vi "Auto 7.vi"(8 "Error In":errorcluster) -> (0 "Error Out":errorcluster)   [LabVIEW 2014]
uses:
  <vilib>/Rock Robotics/WPI/Solenoid/WPI_SolenoidValue.ctl
  <vilib>/Rock Robotics/WPI/Solenoid/WPI_SolenoidSetEnum.vi
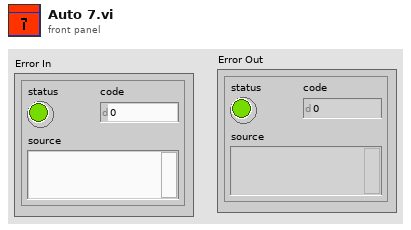
[diagram p1: front panel]
types:
  T1 = typedef "WPI_SolenoidValue.ctl" = enum16{"Off", "On", "Forward", "Reverse"}
  T2 = typedef "WPI_SolenoidDevRef.ctl" = cluster{"DevStatus":errorcluster, "Pneumatics Control Module":u8, "Forward Solenoid Channel":T3, "Reverse Solenoid Channel":T3}
  T3 = typedef "WPI_SolenoidChannel.ctl" = enum8{"Solenoid 0", "Solenoid 1", "Solenoid 2", "Solenoid 3", "Solenoid 4", "Solenoid 5", "Solenoid 6", "Solenoid 7", "Invalid"}
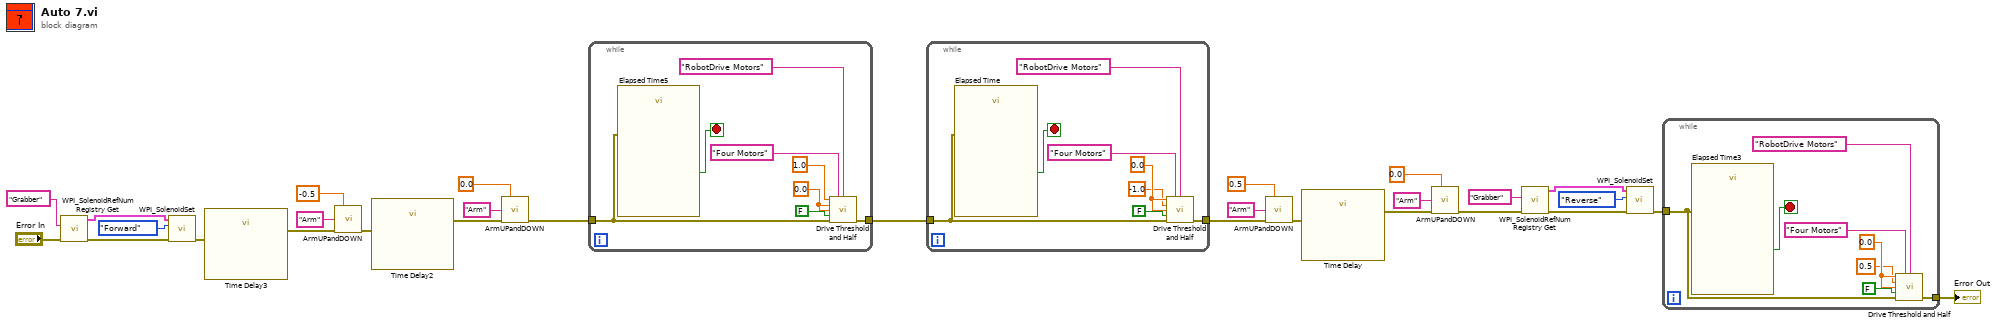
[diagram p0: block diagram]
diagram:
  n1 = call <vilib>:"WPI_SolenoidRefNum Registry Get.vi"("error in (no error)"="Error In", "refnum name"="Grabber") -> ("error out"=w16:errorcluster, "SolenoidDevRef"=w17:T2)  [unwired: 8 in]
  n2 = call-poly <vilib>:"WPI_SolenoidSet.vi"("error in (no error)"=w16, "Value"=WPI_SolenoidValue."Forward", "SolenoidDevRef"=w17) -> ("error out"=w5:errorcluster)  [unwired: 7 in, 1 out]
  n3 = call "Time Delay3"("error in (no error)"=w5) -> ("error out"=w4:errorcluster)  [unwired: 10 in]
  n4 = call "ArmUPandDOWN.vi"("Arm Value"=-0.5, "Arm"="Arm" ("refnum name"), "Error In"=w4) -> ("Error Out"=w27:errorcluster)  [unwired: 12 in]
  n5 = call "Time Delay2"("error in (no error)"=w27) -> ("error out"=w10:errorcluster)  [unwired: 10 in]
  n6 = call "ArmUPandDOWN.vi"("Arm Value"=0.0, "Arm"="Arm" ("refnum name"), "Error In"=w10) -> ("Error Out"=w3:errorcluster)  [unwired: 12 in]
  n7 = while {
    tunnel: w3 -> [w32]
    tunnel: [w34] -> w2
    stop <- w33 stop-if-true
    w30 = 0.0 ("X In")
    n8 = call "Elapsed Time5"("error in (no error)"=w32) -> ("Time has Elapsed"=w33:bool)  [unwired: 11 in, 7 out]
    n9 = call "Drive Threshold and Half.vi"("X In"=1.0 ("Arm Value"), "Drive refnum name"="Four Motors" ("refnum name"), "Send to DB Name"="RobotDrive Motors" ("Name"), "Y In"=w30, "R In"=w30, "Speed Toggle"=FALSE ("Grabber Open/Close"), "Error In"=w32) -> ("Error Out"=w34:errorcluster)  [unwired: 8 in]
  }
  n10 = while {
    tunnel: w2 -> [w38]
    tunnel: [w42] -> w1
    stop <- w39 stop-if-true
    w41 = 0.0 ("Arm Value")
    n11 = call "Elapsed Time"("error in (no error)"=w38) -> ("Time has Elapsed"=w39:bool)  [unwired: 11 in, 7 out]
    n12 = call "Drive Threshold and Half.vi"("X In"=w41, "Drive refnum name"="Four Motors" ("refnum name"), "Send to DB Name"="RobotDrive Motors" ("Name"), "Y In"=-1.0 ("X In"), "R In"=w41, "Speed Toggle"=FALSE ("Grabber Open/Close"), "Error In"=w38) -> ("Error Out"=w42:errorcluster)  [unwired: 8 in]
  }
  n13 = call "ArmUPandDOWN.vi"("Arm Value"=0.5, "Arm"="Arm" ("refnum name"), "Error In"=w1) -> ("Error Out"=w25:errorcluster)  [unwired: 12 in]
  n14 = call "Time Delay"("error in (no error)"=w25) -> ("error out"=w7:errorcluster)  [unwired: 10 in]
  n15 = call "ArmUPandDOWN.vi"("Arm Value"=0.0, "Arm"="Arm" ("refnum name"), "Error In"=w7) -> ("Error Out"=w6:errorcluster)  [unwired: 12 in]
  n16 = call <vilib>:"WPI_SolenoidRefNum Registry Get.vi"("error in (no error)"=w6, "refnum name"="Grabber") -> ("error out"=w21:errorcluster, "SolenoidDevRef"=w22:T2)  [unwired: 8 in]
  n17 = call-poly <vilib>:"WPI_SolenoidSet.vi"("error in (no error)"=w21, "Value"=WPI_SolenoidValue."Reverse", "SolenoidDevRef"=w22) -> ("error out"=w18:errorcluster)  [unwired: 7 in, 1 out]
  n18 = while {
    tunnel: w18 -> [w46]
    tunnel: [w50] -> w26
    stop <- w47 stop-if-true
    w49 = 0.0 ("Arm Value")
    n19 = call "Elapsed Time3"("error in (no error)"=w46) -> ("Time has Elapsed"=w47:bool)  [unwired: 11 in, 7 out]
    n20 = call "Drive Threshold and Half.vi"("X In"=w49, "Drive refnum name"="Four Motors" ("refnum name"), "Send to DB Name"="RobotDrive Motors" ("Name"), "Y In"=0.5 ("X In"), "R In"=w49, "Speed Toggle"=FALSE ("Grabber Open/Close"), "Error In"=w46) -> ("Error Out"=w50:errorcluster)  [unwired: 8 in]
  }
  "Error Out" <- w26
